vi "System1.vi"() -> ()   [LabVIEW 2015]
uses:
  <vilib>/DAQmx/write.llb/DAQmx Write (Digital 1D Bool NChan 1Samp 1Line).vi
  <vilib>/DAQmx/write.llb/DAQmx Write (Analog DBL 1Chan 1Samp).vi
  <vilib>/Analysis/baseanly.llb/Mean (DBL).vi
  <vilib>/DAQmx/read.llb/DAQmx Read (Analog 1D Wfm NChan NSamp).vi
  <vilib>/DAQmx/miscellaneous.llb/DAQmx Fill In Error Info.vi
  <vilib>/addons/control/pid/NI_PID_autopid.lvlib
  <vilib>/Analysis/NI_AALBase.lvlib
panel:
  in  "On/Off":bool
  in  "Stop All":bool
  in  "Manual Control 2":bool
  in  "Voltage setting 2":dbl format="%#_13g"
  out "Voltage Reading(pressure) 2":dbl format="%#_13g"
  out "Pressure 2":dbl format="%#.3g"
  out "Pressure Chart 2":dbl(graph)
  in  "autotuning parameters 2":T1={"controller type"=1, "relay cycles"=3, "relay amplitude"=1.0, "control specification"=2, "PV noise level"=0.1} {"PV noise level" format="%.2f"; "control specification" items=["normal", "fast", "slow"]; "relay amplitude" format="%.2f"; "controller type" items=["PID", "PI", "P"]}
  in  "PID gains 2":T2={"proportional gain (Kc)"=1.0, "integral time (Ti, min)"=0.01, "derivative time (Td, min)"=0.0} {"derivative time (Td, min)" format="%.3f"; "integral time (Ti, min)" format="%.3f"; "proportional gain (Kc)" format="%.3f"}
  out "PID gains out 2":T2={"proportional gain (Kc)"=1.0, "integral time (Ti, min)"=0.01, "derivative time (Td, min)"=0.0} {"derivative time (Td, min)" format="%.3f"; "integral time (Ti, min)" format="%.3f"; "proportional gain (Kc)" format="%.3f"}
  in  "autotune? (F) 2":bool
  in  "reinitialize? (F) 2":bool
  in  "setpoint in Bar 2":dbl format="%#.5f"
  out "Control Value 2":dbl
  in  "Voltage setting":dbl format="%#_13g"
  in  "Manual Control":bool
  out "Control Value":dbl
  in  "setpoint in Bar":dbl format="%#.5f"
  in  "reinitialize? (F)":bool
  in  "autotune? (F)":bool
  out "PID gains out":T2={"proportional gain (Kc)"=1.0, "integral time (Ti, min)"=0.01, "derivative time (Td, min)"=0.0} {"derivative time (Td, min)" format="%.3f"; "integral time (Ti, min)" format="%.3f"; "proportional gain (Kc)" format="%.3f"}
  in  "PID gains":T2={"proportional gain (Kc)"=1.0, "integral time (Ti, min)"=0.01, "derivative time (Td, min)"=0.0} {"derivative time (Td, min)" format="%.3f"; "integral time (Ti, min)" format="%.3f"; "proportional gain (Kc)" format="%.3f"}
  in  "autotuning parameters":T1={"controller type"=1, "relay cycles"=3, "relay amplitude"=1.0, "control specification"=2, "PV noise level"=0.1} {"PV noise level" format="%.2f"; "control specification" items=["normal", "fast", "slow"]; "relay amplitude" format="%.2f"; "controller type" items=["PID", "PI", "P"]}
  out "Pressure Chart":dbl(graph)
  out "Pressure":dbl format="%#.3g"
  out "Voltage Reading(pressure)":dbl format="%#_13g"
  # "Pressure Vessel 2"
  # "Pressure Vessel 1"
  # "Readings"
  # "Controls"
  # "Readings"
  # "Controls"
  # "PID Settings"
  # "51.12139\n\n0.044676"
  # "Valves"
  # "Pump 3"
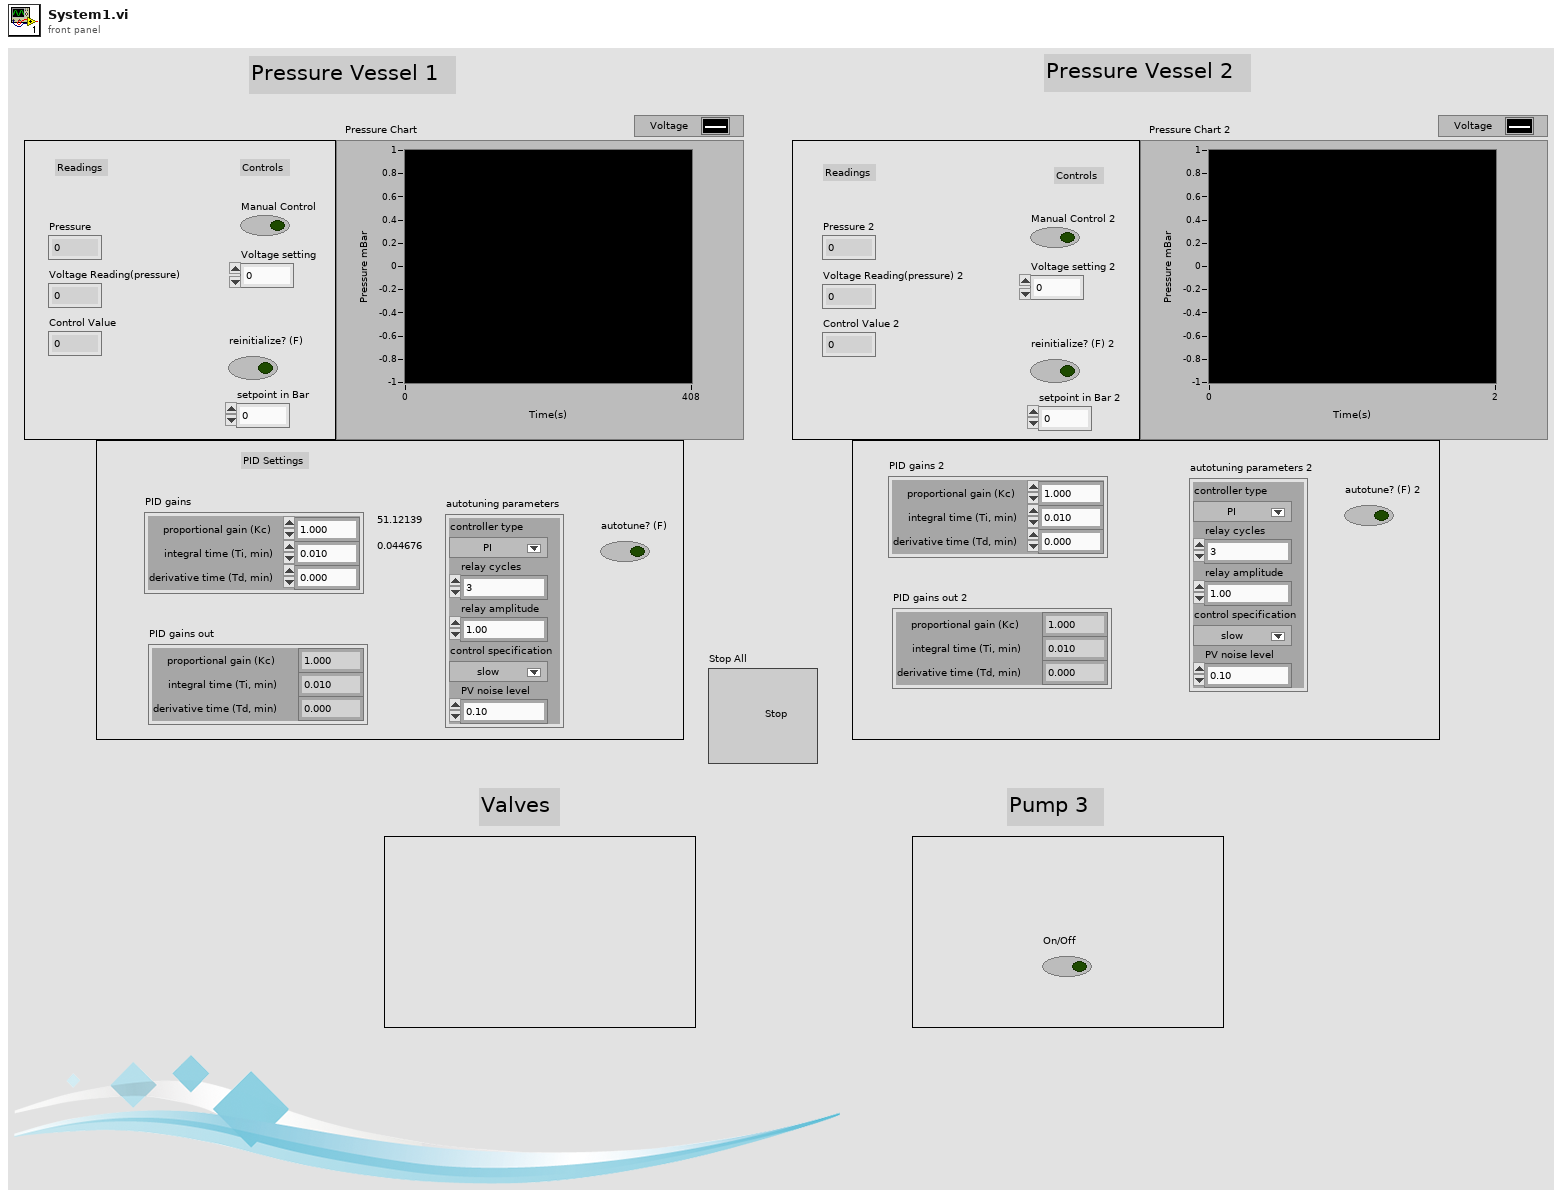
[diagram p1: front panel]
types:
  T1 = cluster{"controller type":u16, "relay cycles":i32, "relay amplitude":dbl, "control specification":u16, "PV noise level":dbl}
  T2 = cluster{"proportional gain (Kc)":dbl, "integral time (Ti, min)":dbl, "derivative time (Td, min)":dbl}
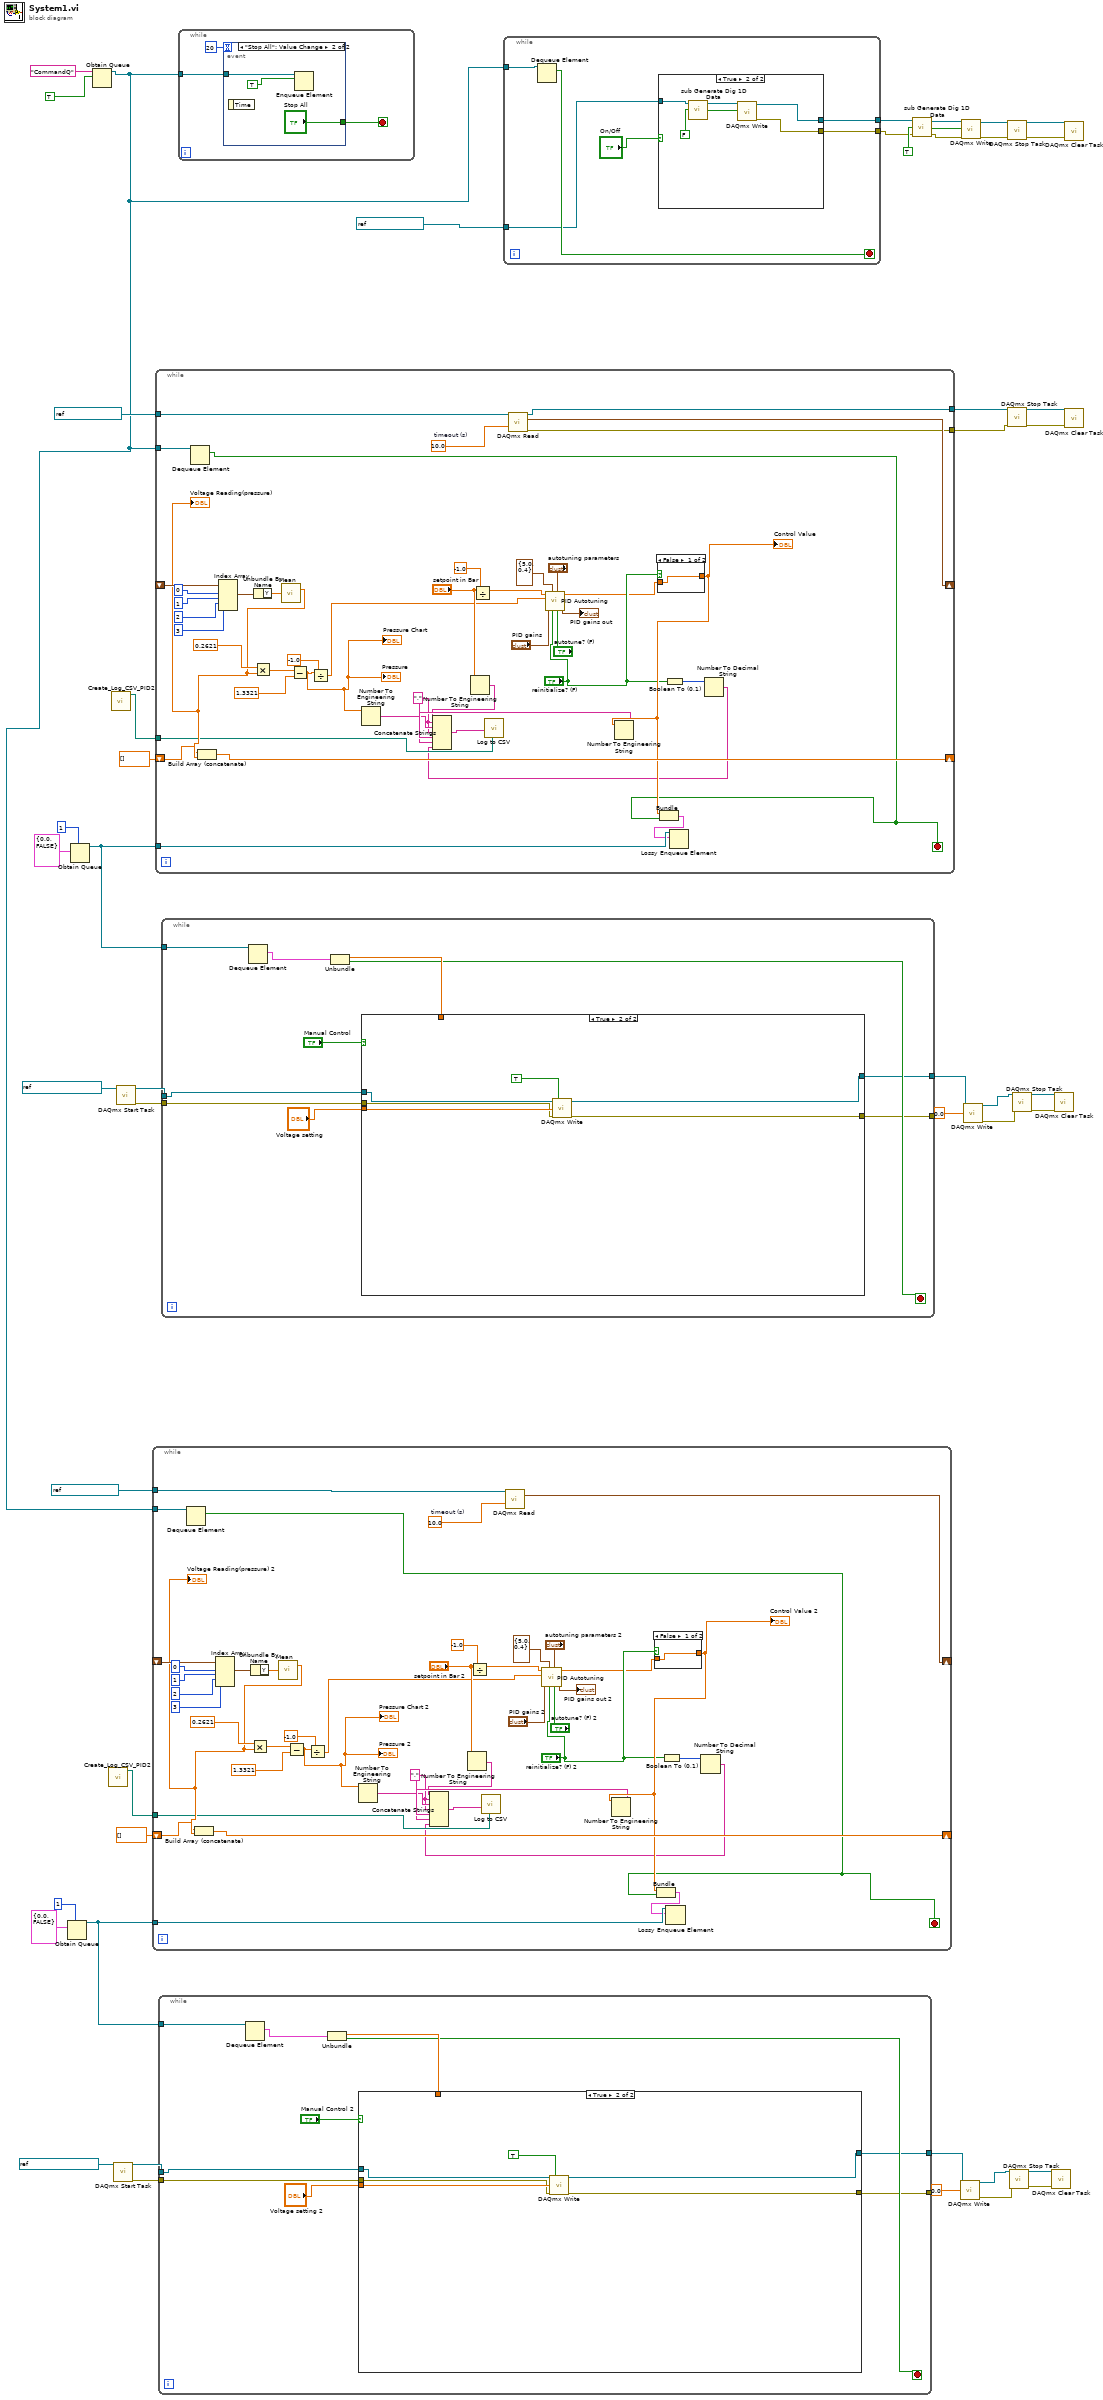
[diagram p0: block diagram]
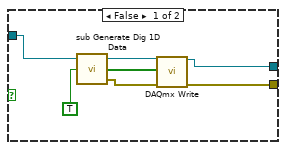
[diagram p2: hidden frame]
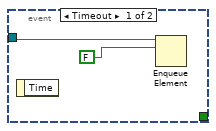
[diagram p3: hidden frame]
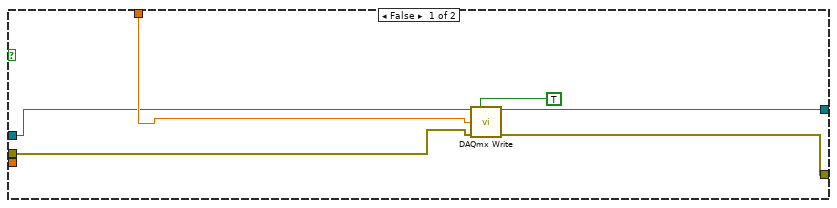
[diagram p4: hidden frame]
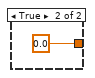
[diagram p5: hidden frame]
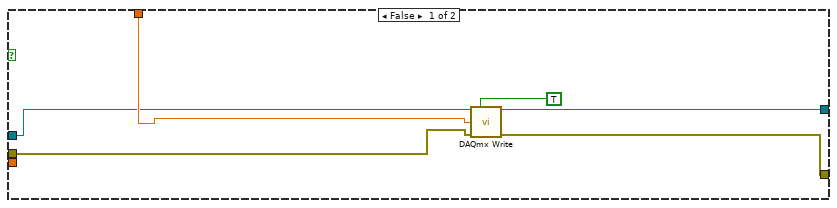
[diagram p6: hidden frame]
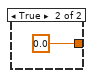
[diagram p7: hidden frame]
diagram:
  n1 = Obtain Queue(max queue size (-1, unlimited)=1, element data type=cluster{dbl, bool} {0.0, FALSE}) -> (queue out=w31:refnum<queue>)  [unwired: 3 in, 2 out]
  n2 = Obtain Queue(max queue size (-1, unlimited)=1, element data type=cluster{dbl, bool} {0.0, FALSE}) -> (queue out=w46:refnum<queue>)  [unwired: 3 in, 2 out]
  n3 = Obtain Queue(name (unnamed)="CommandQ", element data type=TRUE) -> (queue out=w16:refnum<queue>)  [unwired: 3 in, 2 out]
  n4 = call "Create_Log_CSV_PID2.vi"() -> ("path"=w27:path)  [unwired: 11 in]
  n5 = call "Create_Log_CSV_PID2.vi"() -> ("path"=w42:path)  [unwired: 11 in]
  n6 = call <vilib>:"DAQmx Start Task.vi"("task/channels in"=refnum<k21> "MyVoltageOutTask") -> ("task out"=w26:refnum<k21>, "error out"=w25:errorcluster)  [unwired: 13 in]
  n7 = call <vilib>:"DAQmx Start Task.vi"("task/channels in"=refnum<k21> "MyVoltageOutTask") -> ("task out"=w41:refnum<k21>, "error out"=w40:errorcluster)  [unwired: 13 in]
  n8 = while {
    tunnel: refnum<k21> "MyVoltageTask" -> [w86]
    shift-right: [w80] -> _
    shift-left: _ -> [w73]
    tunnel: w31 -> [w79]
    shift-right: [w68] -> _
    shift-left: dbl[] [] -> [w69]
    tunnel: w27 -> [w62]
    tunnel: w16 -> [w50]
    stop <- w49 stop-if-true
    w57 = ","
    w90 = 10.0  # timeout (s)
    n9 = Dequeue Element(queue=w50) -> (element=w49:bool)  [unwired: 2 in, 3 out]
    n10 = Index Array(array=w73, index #1=0 ("index"), index #2=1 ("index"), index #3=2 ("index"), index #4=3 ("index")) -> (element #1=w72:waveform(dbl))  [unwired: 3 out]
    n11 = Unbundle By Name(w72) -> ("Y"=w71:dbl[])
    n12 = call-poly <vilib>:"Mean.vi"("X"=w71) -> ("mean"=w70:dbl)  [unwired: 1 out]
    "Voltage Reading(pressure) 2" <- w70
    n13 = Build Array (concatenate)(w69, w70) -> (w68:dbl[])
    n14 = Multiply(x=0.2621, y=w70) -> (x*y=w88:dbl)
    n15 = Subtract(x=w88, y=1.3321) -> (x-y=w66:dbl)
    "Pressure 2" <- w66
    "Pressure Chart 2" <- w66
    n16 = Divide(x=w66, y=-1.0) -> (x/y=w54:dbl)
    n17 = Number To Engineering String(4:w66) -> (0:w61:string)  [unwired: 3 in]
    n18 = Number To Engineering String(4:"setpoint in Bar 2") -> (0:w60:string)  [unwired: 3 in]
    n19 = Divide(x="setpoint in Bar 2", y=-1.0) -> (x/y=w53:dbl)
    n20 = call-poly <vilib>:"DAQmx Read.vi"("task/channels in"=w86, "timeout"=w90) -> ("data"=w80:waveform(dbl)[])  [unwired: 11 in, 2 out]
    n21 = call <vilib>:"PID Autotuning.vi"("autotune? (F)"="autotune? (F) 2", "autotuning parameters"="autotuning parameters 2", "reinitialize? (F)"="reinitialize? (F) 2", "output range"=cluster{"output high":dbl, "output low":dbl} {"output high"=5.0, "output low"=0.4}, "PID gains"="PID gains 2", "process variable"=w54, "setpoint"=w53) -> ("PID gains out"=→"PID gains out 2":T2, "output"=w51:dbl)  [unwired: 1 in, 2 out]
    n22 = case shown="False" "reinitialize? (F) 2" {
      tunnel: [w91 0.0] -> w65
      tunnel: w51 -> [w91 _]
      frame False {
      }
      frame True {
      }
    }
    "Control Value 2" <- w65
    n23 = Number To Engineering String(4:w65) -> (0:w64:string)  [unwired: 3 in]
    n24 = Bundle("output"=w65, w49) -> (w78:cluster{"output":dbl, bool})  [unwired: 1 in]
    n25 = Boolean To (0,1)(Boolean="reinitialize? (F) 2") -> (0, 1=w58:i16)
    n26 = Lossy Enqueue Element(queue=w79, element=w78) -> ()  [unwired: 1 in, 4 out]
    n27 = Number To Decimal String(number=w58) -> (decimal integer string=w56:string)  [unwired: 1 in]
    n28 = Concatenate Strings(w60, w57, w61, w57, w64, w57, w56) -> (w63:string)
    n29 = call "Log to CSV.vi"("Data Str"=w63, "Path"=w62) -> ()  [unwired: 5 in, 1 out]
  }
  n30 = while {
    tunnel: refnum<k21> "MyVoltageTask" -> [w132]
    shift-right: [w126] -> _
    shift-left: _ -> [w119]
    tunnel: w46 -> [w125]
    shift-right: [w114] -> _
    shift-left: dbl[] [] -> [w115]
    tunnel: w42 -> [w108]
    tunnel: w16 -> [w96]
    tunnel: [w94] -> w2
    tunnel: [w93] -> w1
    stop <- w95 stop-if-true
    w103 = ","
    w136 = 10.0  # timeout (s)
    n31 = Dequeue Element(queue=w96) -> (element=w95:bool)  [unwired: 2 in, 3 out]
    n32 = Index Array(array=w119, index #1=0 ("index"), index #2=1 ("index"), index #3=2 ("index"), index #4=3 ("index")) -> (element #1=w118:waveform(dbl))  [unwired: 3 out]
    n33 = Unbundle By Name(w118) -> ("Y"=w117:dbl[])
    n34 = call-poly <vilib>:"Mean.vi"("X"=w117) -> ("mean"=w116:dbl)  [unwired: 1 out]
    "Voltage Reading(pressure)" <- w116
    n35 = Build Array (concatenate)(w115, w116) -> (w114:dbl[])
    n36 = Multiply(x=0.2621, y=w116) -> (x*y=w134:dbl)
    n37 = Subtract(x=w134, y=1.3321) -> (x-y=w112:dbl)
    "Pressure" <- w112
    "Pressure Chart" <- w112
    n38 = Divide(x=w112, y=-1.0) -> (x/y=w100:dbl)
    n39 = Number To Engineering String(4:w112) -> (0:w107:string)  [unwired: 3 in]
    n40 = Number To Engineering String(4:"setpoint in Bar") -> (0:w106:string)  [unwired: 3 in]
    n41 = Divide(x="setpoint in Bar", y=-1.0) -> (x/y=w99:dbl)
    n42 = call-poly <vilib>:"DAQmx Read.vi"("task/channels in"=w132, "timeout"=w136) -> ("task out"=w94:refnum<k21>, "data"=w126:waveform(dbl)[], "error out"=w93:errorcluster)  [unwired: 11 in]
    n43 = call <vilib>:"PID Autotuning.vi"("autotune? (F)"="autotune? (F)", "autotuning parameters"="autotuning parameters", "reinitialize? (F)"="reinitialize? (F)", "output range"=cluster{"output high":dbl, "output low":dbl} {"output high"=5.0, "output low"=0.4}, "PID gains"="PID gains", "process variable"=w100, "setpoint"=w99) -> ("PID gains out"=→"PID gains out":T2, "output"=w97:dbl)  [unwired: 1 in, 2 out]
    n44 = case shown="False" "reinitialize? (F)" {
      tunnel: [w137 0.0] -> w111
      tunnel: w97 -> [w137 _]
      frame False {
      }
      frame True {
      }
    }
    "Control Value" <- w111
    n45 = Number To Engineering String(4:w111) -> (0:w110:string)  [unwired: 3 in]
    n46 = Bundle("output"=w111, w95) -> (w124:cluster{"output":dbl, bool})  [unwired: 1 in]
    n47 = Boolean To (0,1)(Boolean="reinitialize? (F)") -> (0, 1=w104:i16)
    n48 = Lossy Enqueue Element(queue=w125, element=w124) -> ()  [unwired: 1 in, 4 out]
    n49 = Number To Decimal String(number=w104) -> (decimal integer string=w102:string)  [unwired: 1 in]
    n50 = Concatenate Strings(w106, w103, w107, w103, w110, w103, w102) -> (w109:string)
    n51 = call "Log to CSV.vi"("Data Str"=w109, "Path"=w108) -> ()  [unwired: 5 in, 1 out]
  }
  n52 = while {
    tunnel: w31 -> [w148]
    tunnel: w26 -> [w146]
    tunnel: [w141] -> w23
    tunnel: w25 -> [w140]
    tunnel: [w139] -> _
    stop <- w142 stop-if-true
    n53 = Dequeue Element(queue=w148) -> (element=w145:cluster{dbl, bool})  [unwired: 2 in, 3 out]
    n54 = Unbundle(w145) -> (w144:dbl, w142:bool)
    n55 = case shown="True" "Manual Control 2" {
      tunnel: w146 -> [w152 w159]
      tunnel: w144 -> [w153 _]
      tunnel: "Voltage setting 2" -> [_ w158]
      tunnel: [w151 w157] -> w141
      tunnel: w140 -> [w150 w156]
      tunnel: [w149 w155] -> w139
      frame False {
        n56 = call-poly <vilib>:"DAQmx Write.vi"("task/channels in"=w152, "auto start"=TRUE, "data"=w153, "error in"=w150) -> ("task out"=w151:refnum<k21>, "error out"=w149:errorcluster)  [unwired: 9 in, 1 out]
      }
      frame True {
        n57 = call-poly <vilib>:"DAQmx Write.vi"("task/channels in"=w159, "auto start"=TRUE, "data"=w158, "error in"=w156) -> ("task out"=w157:refnum<k21>, "error out"=w155:errorcluster)  [unwired: 9 in, 1 out]
      }
    }
  }
  n58 = while {
    tunnel: w46 -> [w170]
    tunnel: w41 -> [w168]
    tunnel: [w163] -> w38
    tunnel: w40 -> [w162]
    tunnel: [w161] -> _
    stop <- w164 stop-if-true
    n59 = Dequeue Element(queue=w170) -> (element=w167:cluster{dbl, bool})  [unwired: 2 in, 3 out]
    n60 = Unbundle(w167) -> (w166:dbl, w164:bool)
    n61 = case shown="True" "Manual Control" {
      tunnel: w168 -> [w174 w181]
      tunnel: w166 -> [w175 _]
      tunnel: "Voltage setting" -> [_ w180]
      tunnel: [w173 w179] -> w163
      tunnel: w162 -> [w172 w178]
      tunnel: [w171 w177] -> w161
      frame False {
        n62 = call-poly <vilib>:"DAQmx Write.vi"("task/channels in"=w174, "auto start"=TRUE, "data"=w175, "error in"=w172) -> ("task out"=w173:refnum<k21>, "error out"=w171:errorcluster)  [unwired: 9 in, 1 out]
      }
      frame True {
        n63 = call-poly <vilib>:"DAQmx Write.vi"("task/channels in"=w181, "auto start"=TRUE, "data"=w180, "error in"=w178) -> ("task out"=w179:refnum<k21>, "error out"=w177:errorcluster)  [unwired: 9 in, 1 out]
      }
    }
  }
  n64 = while {
    tunnel: w16 -> [w184]
    stop <- w183 stop-if-true
    n65 = event shown="[1] \"Stop All\": Value Change" {
      selector: _ -> [_ _]
      dyn-events: _ -> [_ _]
      timeout: 20 -> [_ _]
      tunnel: w184 -> [w186 w190]
      tunnel: [_ "Stop All"] -> w183
      event Timeout {
        n66 = event-data() -> ()  [unwired: 1 in, 1 out]
        n67 = Enqueue Element(queue=w186, element=FALSE) -> ()  [unwired: 2 in, 3 out]
      }
      event "Stop All": Value Change {
        n68 = event-data() -> ()  [unwired: 1 in, 1 out]
        n69 = Enqueue Element(queue=w190, element=TRUE) -> ()  [unwired: 2 in, 3 out]
      }
    }
  }
  n70 = while {
    tunnel: w16 -> [w196]
    tunnel: refnum<k21> "MyVoltageTask" -> [w193]
    tunnel: [w192] -> w8
    tunnel: [w191] -> w7
    stop <- w195 stop-if-true
    n71 = Dequeue Element(queue=w196) -> (element=w195:bool)  [unwired: 2 in, 3 out]
    n72 = case shown="True" "On/Off" {
      tunnel: w193 -> [w200 w209]
      tunnel: [w199 w205] -> w192
      tunnel: [w197 w204] -> w191
      frame False {
        n73 = call <vilib>:"sub Generate Dig 1D Data.vi"("initial value"=TRUE, "task in"=w200) -> ("error out"=w198:errorcluster, "Data"=w202:bool[], "task out"=w201:refnum<k21>)  [unwired: 1 in]
        n74 = call-poly <vilib>:"DAQmx Write.vi"("task/channels in"=w201, "data"=w202, "error in"=w198) -> ("task out"=w199:refnum<k21>, "error out"=w197:errorcluster)  [unwired: 10 in, 1 out]
      }
      frame True {
        n75 = call <vilib>:"sub Generate Dig 1D Data.vi"("initial value"=FALSE, "task in"=w209) -> ("Data"=w207:bool[], "task out"=w208:refnum<k21>)  [unwired: 1 in, 1 out]
        n76 = call-poly <vilib>:"DAQmx Write.vi"("task/channels in"=w208, "data"=w207) -> ("task out"=w205:refnum<k21>, "error out"=w204:errorcluster)  [unwired: 11 in, 1 out]
      }
    }
  }
  n77 = call <vilib>:"sub Generate Dig 1D Data.vi"("error in"=w7, "initial value"=TRUE, "task in"=w8) -> ("error out"=w12:errorcluster, "Data"=w10:bool[], "task out"=w11:refnum<k21>)
  n78 = call-poly <vilib>:"DAQmx Write.vi"("task/channels in"=w23, "data"=0.0) -> ("task out"=w22:refnum<k21>, "error out"=w21:errorcluster)  [unwired: 11 in, 1 out]
  n79 = call-poly <vilib>:"DAQmx Write.vi"("task/channels in"=w11, "data"=w10, "error in"=w12) -> ("task out"=w6:refnum<k21>, "error out"=w5:errorcluster)  [unwired: 10 in, 1 out]
  n80 = call-poly <vilib>:"DAQmx Write.vi"("task/channels in"=w38, "data"=0.0) -> ("task out"=w37:refnum<k21>, "error out"=w36:errorcluster)  [unwired: 11 in, 1 out]
  n81 = call <vilib>:"DAQmx Stop Task.vi"("task/channels in"=w6, "error in"=w5) -> ("task out"=w14:refnum<k21>, "error out"=w13:errorcluster)  [unwired: 12 in]
  n82 = call <vilib>:"DAQmx Stop Task.vi"("task/channels in"=w2, "error in"=w1) -> ("task out"=w3:refnum<k21>, "error out"=w4:errorcluster)  [unwired: 12 in]
  n83 = call <vilib>:"DAQmx Stop Task.vi"("task/channels in"=w22, "error in"=w21) -> ("task out"=w24:refnum<k21>, "error out"=w20:errorcluster)  [unwired: 12 in]
  n84 = call <vilib>:"DAQmx Stop Task.vi"("task/channels in"=w37, "error in"=w36) -> ("task out"=w39:refnum<k21>, "error out"=w35:errorcluster)  [unwired: 12 in]
  n85 = call <vilib>:"DAQmx Clear Task.vi"("task in"=w24, "error in"=w20) -> ()  [unwired: 13 in, 1 out]
  n86 = call <vilib>:"DAQmx Clear Task.vi"("task in"=w39, "error in"=w35) -> ()  [unwired: 13 in, 1 out]
  n87 = call <vilib>:"DAQmx Clear Task.vi"("task in"=w14, "error in"=w13) -> ()  [unwired: 13 in, 1 out]
  n88 = call <vilib>:"DAQmx Clear Task.vi"("task in"=w3, "error in"=w4) -> ()  [unwired: 13 in, 1 out]
